vi "Example Read Callback - FrameRead Callback.vi"(4 "FrameRead":refnum<user-event>, 5 "Event Data":T1, 6 "Control Ref":refnum<k24>, 7 "Event Common Data":T2) -> ()   [LabVIEW 2010]
uses:
  C:/tf/play/labview/Tinkerforge.dll
  Tinkerforge.dll
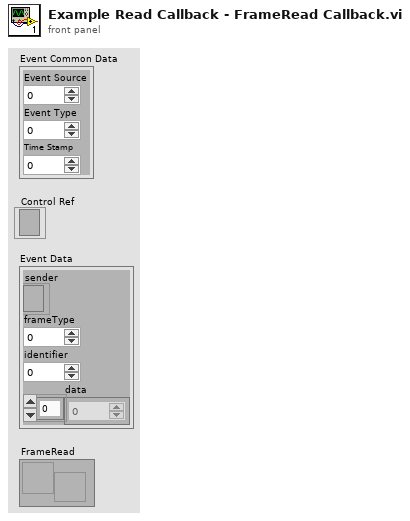
[diagram p1: front panel]
types:
  T1 = cluster{"sender":refnum<k24>, "frameType":u8, "identifier":i64, "data":u8[]}
  T2 = cluster{"Event Source":i32, "Event Type":u32, "Time Stamp":u32}
  T3 = cluster{"data":u8[], "frameType":u8, "identifier":i64}
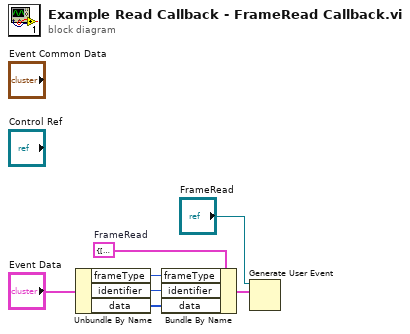
[diagram p0: block diagram]
diagram:
  w6 = T3 {"data"=[], "frameType"=0, "identifier"=0}  # FrameRead
  n1 = Unbundle By Name("Event Data") -> ("frameType"=w5:u8, "identifier"=w4:i64, "data"=w3:u8[])
  n2 = Bundle By Name(cluster=w6, "frameType"=w5, "identifier"=w4, "data"=w3) -> (w2:T3)
  n3 = Generate User Event(user event="FrameRead", event data cluster=w2) -> ()  [unwired: 1 in, 2 out]
